vi "Configure Power Analysis (Power Supply Rejection Ratio).vi"(7 "Vertical Scale (100)":dbl=100.0, 8 "error in (no error)":errorcluster, 9 "End Sweep Frequency (100000 Hz)":i32(ring)=100000 items=["10"=10, "100"=100, "1000"=1000, "10000"=10000, "100000"=100000, "1000000"=1000000, "10000000"=10000000, "20000000"=20000000], 10 "Start Sweep Frequency (100 Hz)":i32(ring)=100 items=["1"=1, "10"=10, "100"=100, "1000"=1000, "10000"=10000, "100000"=100000, "1000000"=1000000, "10000000"=10000000], 11 "VISA resource name":refnum<visa-resource-name>) -> (0 "error out":errorcluster, 3 "VISA resource name out":refnum<visa-resource-name>)   [LabVIEW 2016, in "Agilent 2000 3000 X-Series.lvlib"]
doc: "Configures the power supply rejection ratio (PSRR) analysis.\n\n<B>Note(s):</B>\nThe Power Supply Rejection Ratio (PSRR) test is used to determine how well a voltage regulator rejects ripple noise over different frequency range.\n\nThis analysis provides a signal from the oscilloscope's waveform generator that sweeps its frequency. This signal is used to inject ripple to the DC voltage that feeds the voltage regulator.\n\nThe AC RMS ratio of the input over the output is measured and is plotted over the range of frequencies."
uses:
  Agilent 2000 3000 X-Series.lvlib
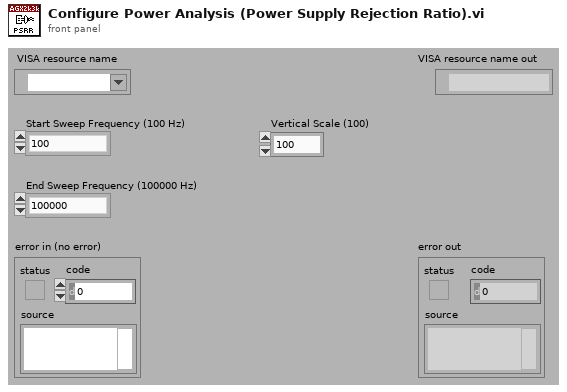
[diagram p1: front panel]
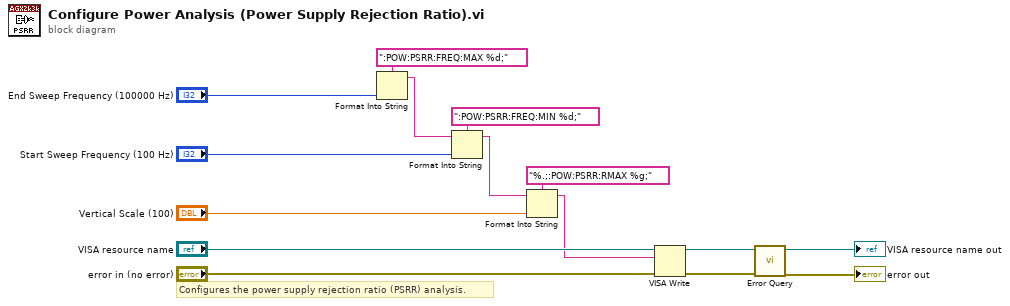
[diagram p0: block diagram]
diagram:
  # "Configures the power supply rejection ratio (PSRR) analysis."
  n1 = Format Into String(format string=":POW:PSRR:FREQ:MAX %d;", "End Sweep Frequency (100000 Hz)") -> (resulting string=w13:string)  [unwired: 2 in, 1 out]
  n2 = Format Into String(format string=":POW:PSRR:FREQ:MIN %d;", initial string=w13, "Start Sweep Frequency (100 Hz)") -> (resulting string=w10:string)  [unwired: 1 in, 1 out]
  n3 = Format Into String(format string="%.;:POW:PSRR:RMAX %g;", initial string=w10, "Vertical Scale (100)") -> (resulting string=w1:string)  [unwired: 1 in, 1 out]
  n4 = VISA Write(VISA resource name="VISA resource name", write buffer=w1, error in (no error)="error in (no error)") -> (VISA resource name out=w5:refnum<visa-resource-name>, error out=w4:errorcluster)  [unwired: 1 out]
  n5 = call "Error Query.vi"("error in (no error)"=w4, "VISA resource name"=w5) -> ("error out"=→"error out":errorcluster, "VISA resource name out"=→"VISA resource name out":refnum<visa-resource-name>)  [unwired: 8 out]
